vi "Select Category by Name.vi"(8 "error in (no error)":errorcluster, 10 "Category Name":string, 11 "Database in":refnum<class "Database.lvclass">) -> (0 "error out":errorcluster, 1 "Found?":bool, 2 "Category":refnum<class "Category.lvclass">, 3 "Database out":refnum<class "Database.lvclass">)   [LabVIEW 2018, in "Database.lvclass"]
uses:
  Database.lvclass
  Category/Category.lvclass
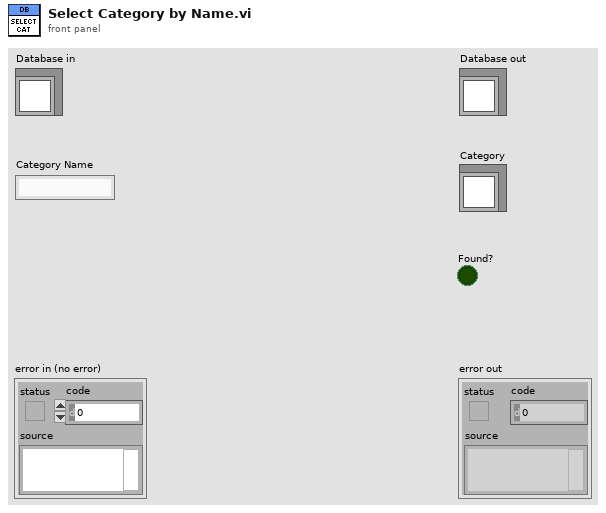
[diagram p1: front panel]
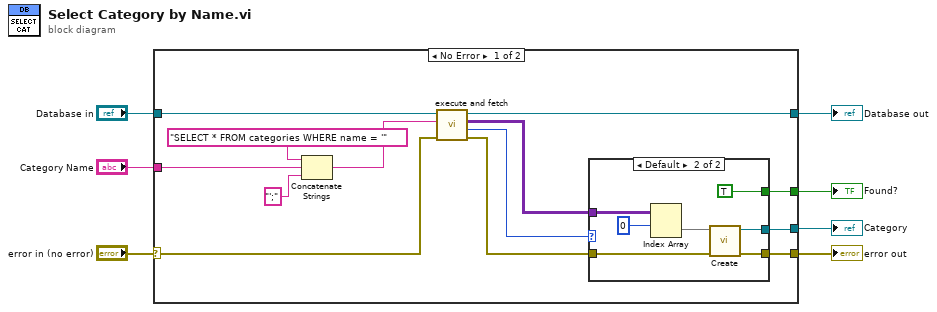
[diagram p0: block diagram]
diagram:
  n1 = case shown="No Error" "error in (no error)" {
    selector: "error in (no error)" -> [w14 w29]
    tunnel: "Database in" -> [w17 w30]
    tunnel: [w16 w30] -> w6
    tunnel: "Category Name" -> [w15 _]
    tunnel: [w12 w29] -> w4
    tunnel: [w10 _] -> w2
    tunnel: [w8 _] -> w1
    frame No Error {
      n2 = Concatenate Strings("SELECT * FROM categories WHERE name = '", w15, "';") -> (w18:string)
      n3 = call "execute and fetch.vi"("error in (no error)"=w14, "SQL query"=w18, "Database in"=w17) -> ("error out"=w13:errorcluster, "Num records"=w9:i32, "recordset data"=w11:variant[][], "Database out"=w16:refnum<class "Database.lvclass">)  [unwired: 5 in]
      n4 = case shown="Default" w9 {
        tunnel: w13 -> [w21 w28]
        tunnel: [w21 w27] -> w12
        tunnel: w11 -> [_ w26]
        tunnel: [_ w23] -> w10
        tunnel: [_ TRUE] -> w8
        frame 0 {
        }
        frame Default {
          n5 = Index Array(array=w26, index (row)=0) -> (element=w24:variant[])  [unwired: 1 in]
          n6 = call "Create.vi"("error in (no error)"=w28, "Record"=w24) -> ("error out"=w27:errorcluster, "Category out"=w23:refnum<class "Category.lvclass">)  [unwired: 8 in]
        }
      }
    }
    frame Error {
    }
  }
  "error out" <- w4
  "Database out" <- w6
  "Category" <- w2
  "Found?" <- w1
